vi "z encoding to string.vi"(8 "error in (no error)":errorcluster, 10 "out_str":cluster{}, 11 "this_":cluster{}) -> (0 "error out":errorcluster, 2 "out_str out":cluster{})   [LabVIEW 2021, in "zenohc.lvlib"]
doc: "void z_encoding_to_string(const struct z_loaned_encoding_t *this_,\n struct z_owned_string_t *out_str);"
uses:
  zenohc.lvlib
  zenohc.dll
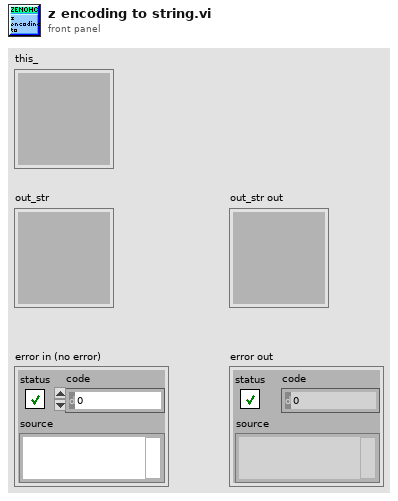
[diagram p1: front panel]
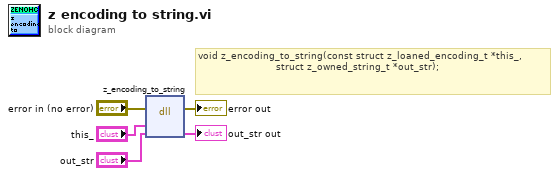
[diagram p0: block diagram]
diagram:
  # "void z_encoding_to_string(const struct z_loaned_encoding_t *this_,\n                          struct z_owned_string_t *out_str);"
  n1 = dll-call lib="D:/dev/zenoh_labview/zenohc/zenohc.*" fn="z_encoding_to_string"(error in="error in (no error)", "this_"="this_", "out_str"="out_str") -> (error out=→"error out":errorcluster, "out_str"=→"out_str out":cluster{})  [unwired: 4 in, 1 out]
